vi "Data Server Encode Response Filename.vi"(6 "FA Stopped?":bool, 8 "error in (no error)":errorcluster, 10 "Filename":string, 11 "Time Stamp":timestamp) -> (0 "error out":errorcluster, 3 "Output string":string)   [LabVIEW 2011, in "Data Server VIs.lvlib"]
uses:
  Data Server VIs.lvlib
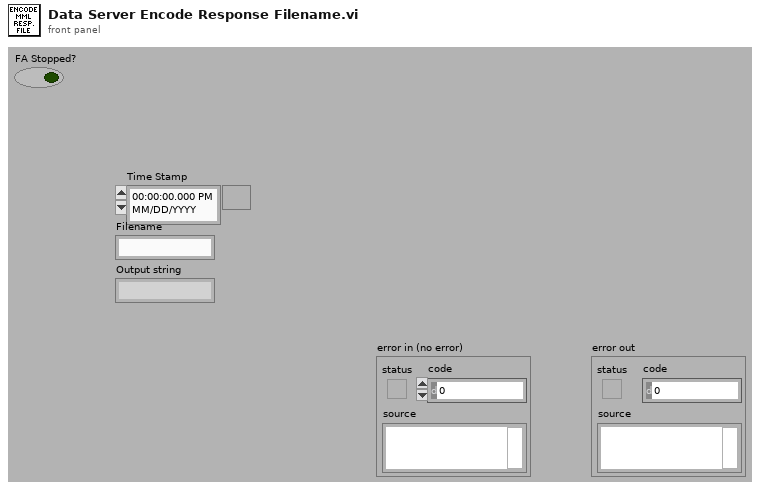
[diagram p1: front panel]
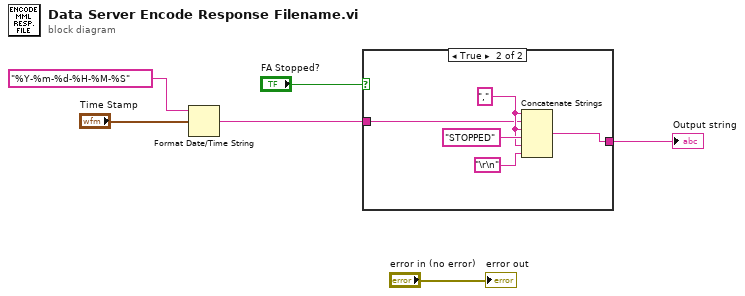
[diagram p0: block diagram]
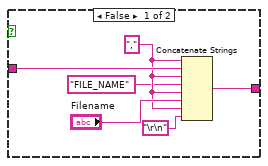
[diagram p2: hidden frame]
diagram:
  n1 = Format Date/Time String(time format string (%c)="%Y-%m-%d-%H-%M-%S", seconds (now)="Time Stamp") -> (date/time string=w4:string)  [unwired: 1 in]
  n2 = case shown="True" "FA Stopped?" {
    tunnel: w4 -> [w12 w14]
    tunnel: [w8 w13] -> w3
    frame False {
      w10 = "," ("string")
      n3 = Concatenate Strings(w10, w12, w10, "FILE_NAME" ("string"), w10, "Filename", w10, "\r\n") -> (w8:string)
    }
    frame True {
      w15 = "," ("string")
      n4 = Concatenate Strings(w15, w14, w15, "STOPPED" ("string"), w15, "\r\n") -> (w13:string)
    }
  }
  "Output string" <- w3
  "error out" <- "error in (no error)"
